vi "Get settings chain.vi"(8 "error in (no error)":errorcluster, 11 "ServiceManagerLoader in":refnum<class "ServiceManagerLoader.lvclass">) -> (0 "error out":errorcluster, 1 "class name":string[](array[string]), 2 "settings":variant[](array[variant]), 3 "ServiceManagerLoader out":refnum<class "ServiceManagerLoader.lvclass">)   [LabVIEW 2012, in "ServiceManagerLoader.lvclass"]
doc: "Returns an array of variants containing the settings clusters of each class in the inheritance chain (lowest child class first), together with an array of all class names in the inheritance chain.\n\nFor classes without settings cluster, the settings chain contains empty variants."
uses:
  ServiceManagerLoader.lvclass
  Murmex/LabVIEW/Murmex/Murmex/Murmex.lvclass
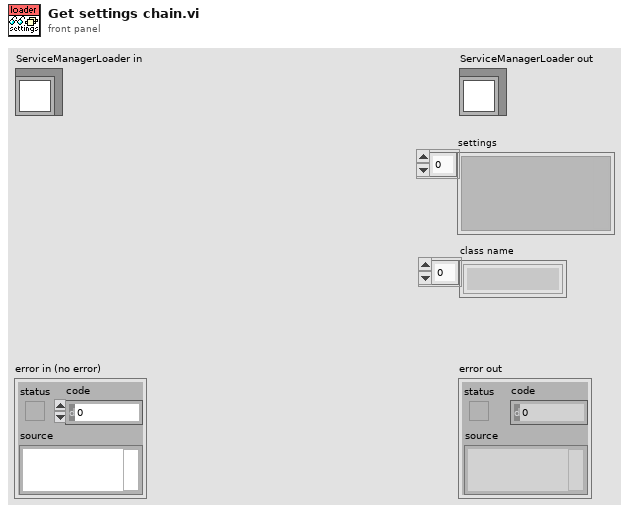
[diagram p1: front panel]
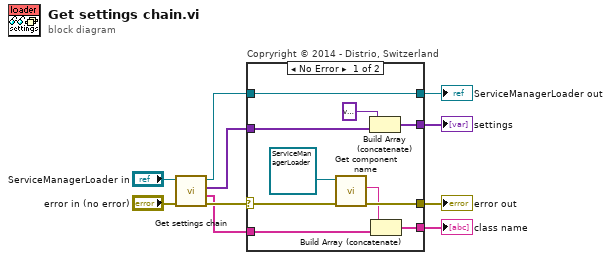
[diagram p0: block diagram]
diagram:
  n1 = call-parent "Get settings chain.vi"("error in (no error)"="error in (no error)", "MurmexBase in"="ServiceManagerLoader in") -> ("error out"=w8:errorcluster, "class name"=w5:string[], "settings"=w6:variant[], "MurmexBase out"=w7:refnum<class "ServiceManagerLoader.lvclass">)  [unwired: 6 in]
  n2 = case "Copryright © 2014 - Distrio, Switzerland" shown="No Error" w8 {
    selector: w8 -> [w19 w22]
    tunnel: [w18 w22] -> w1
    tunnel: [w15 w21] -> w3
    tunnel: w7 -> [w15 w21]
    tunnel: [w20 _] -> w2
    tunnel: [w16 _] -> w4
    tunnel: w6 -> [w13 _]
    tunnel: w5 -> [w11 _]
    frame No Error {
      n3 = call "Get component name.vi"("error in (no error)"=w19, "Murmex in"=refnum<class "ServiceManagerLoader.lvclass"> refnum ("ServiceManagerLoader out")) -> ("error out"=w18:errorcluster, "component name"=w17:string)  [unwired: 7 in, 1 out]
      n4 = Build Array (concatenate)(variant ("Variant"), w13) -> (w20:variant[])
      n5 = Build Array (concatenate)(w17, w11) -> (w16:string[])
    }
    frame Error {
    }
  }
  "error out" <- w1
  "ServiceManagerLoader out" <- w3
  "settings" <- w2
  "class name" <- w4
